vi "dt缩放.vi"() -> ()   [LabVIEW 2018]
uses:
  <vilib>/Waveform/WDTOps.llb/WDT Scale Delta t DBL.vi
  <vilib>/measure/NI_MABase.lvlib
panel:
  in  "scale factor":dbl=1000.0 caption="缩放因子" format="%0.2f"
  out "波形图 2":waveform(dbl)(graph)
  out "波形图":waveform(dbl)(graph)
  in  "停止":bool
  in  "phase":dbl caption="相位" format="%.2p"
  in  "offset":dbl caption="偏移量" format="%0.2p"
  in  "signal type":T1(ring) caption="信号类型"
  in  "amplitude":dbl=1.0 caption="幅值" format="%0.2p"
  in  "frequency":dbl=10.0 caption="频率" format="%0.2p"
  out "字符串":string="dt缩放：\n将波形的dt乘以指定的缩放因子\n该操作会增加或降低波形的采样率"
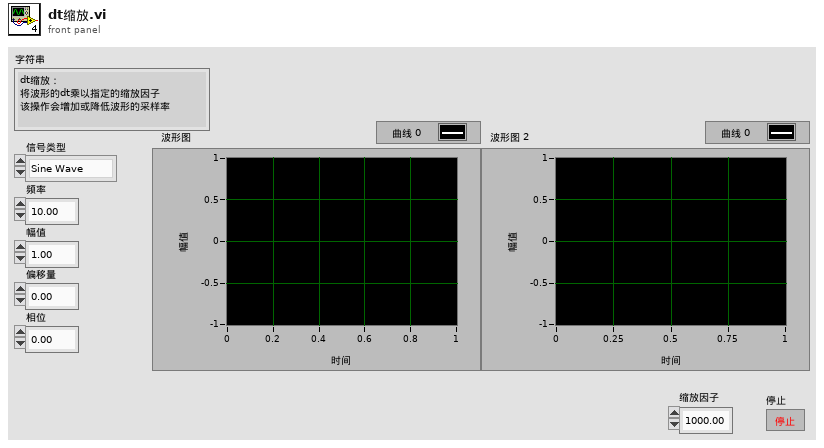
[diagram p1: front panel]
types:
  T1 = enum16{"Sine Wave", "Triangle Wave", "Square Wave", "Sawtooth Wave"}
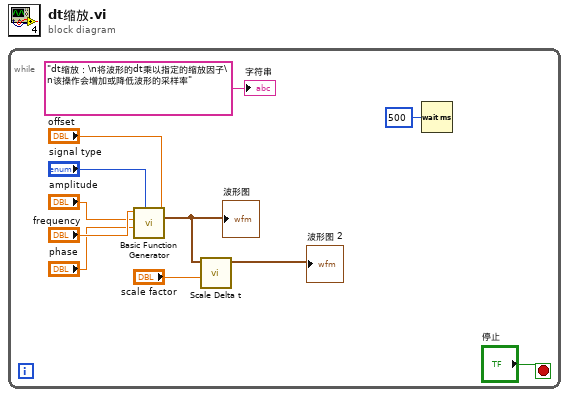
[diagram p0: block diagram]
diagram:
  n1 = while {
    stop <- "停止" stop-if-true
    n2 = call <vilib>:"Basic Function Generator.vi"("offset"="offset", "signal type"="signal type", "phase"="phase", "amplitude"="amplitude", "frequency"="frequency") -> ("signal out"=w4:waveform(dbl))  [unwired: 4 in, 2 out]
    "波形图" <- w4
    n3 = call-poly <vilib>:"Scale Delta t.vi"("scale factor"="scale factor", "waveform in"=w4) -> ("waveform out"=→"波形图 2":waveform(dbl))  [unwired: 8 in, 1 out]
    n4 = Wait (ms)(milliseconds to wait=u32 500 ("等待时间（毫秒）")) -> ()  [unwired: 1 out]
    "字符串" <- "dt缩放：\n将波形的dt乘以指定的缩放因子\n该操作会增加或降低波形的采样率"
  }
